vi "System Monitor.Async.vi"(10 "Parameters":variant, 11 "Process":refnum<class "Process.lvclass">) -> ()   [LabVIEW 2027, in "System Monitor Engine.lvlib"]
uses:
  System Monitor Engine.lvlib
  <vilib>/NI/NIVS Inline Async API/_VS Inline Async API/Process/Process.lvclass
  <vilib>/NI/NIVS Inline Async API/_VS Inline Async API/Process/Process.lvclass/Process.ctl
  Shared/Compiled.Settings.ctl
  Shared/System Monitor Settings.ctl
  <vilib>/Platform/TimedLoop/XDataNode/timing_clust.ctl
  <vilib>/Platform/TimedLoop/XDataNode/nitl_modes.ctl
  <vilib>/Platform/TimedLoop/XDataNode/wakeup.ctl
  <vilib>/NI/NIVS Inline Async API/_Data Access Engine/Access Type Classes/Write/Write.lvclass/Write.ctl
  <vilib>/NI/NIVS Inline Async API/_Data Access Engine/Data Access Engine/Methods/Write.Data.vi
  <vilib>/NI/NIVS Inline Async API/_VS Inline Async API/Error Handling Process/SubVIs/Error.ConvertArray.vi
  <vilib>/NI/NIVS Inline Async API/_Data Access Engine/Access Type Classes/Write/Write.ProcessData.vi
  <vilib>/NI/NIVS Inline Async API/_Data Access Engine/Access Type Classes/Write/Write.Buffer.vi
  <vilib>/NI/NIVS Inline Async API/_Data Access Engine/Access Type Classes/Write/Write.Commit.vi
  Shared/Constants.vi
  <vilib>/NI/NIVS Inline Async API/_Data Access Engine/Data Access Engine/Methods/Write.Lookup.vi
  <vilib>/NI/NIVS Inline Async API/_Data Access Engine/Data Access Engine/Data Access Engine.lvclass
  <vilib>/platform/TimedLoop/XDataNode/XDataNode.xnode
  Shared/System Monitor Shared.lvlib
  <vilib>/NI VeriStand/Custom Device Tools/Custom Device Utility Library/Custom Device Utility Library.lvlib
  <vilib>/Platform/TimedLoop/XDataNode/XDNodeRunTimeDep.lvlib
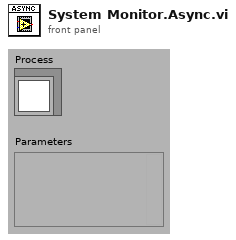
[diagram p1: front panel]
types:
  T1 = typedef "System Monitor Shared.lvlib/Compiled.Settings.ctl" = cluster{"Name":string, "System Monitor Settings":T2}
  T2 = typedef "System Monitor Shared.lvlib/System Monitor Settings.ctl" = cluster{"Number of CPU Cores":u64, "Update Rate (Hz)":dbl}
  T3 = typedef "Data Access Engine.lvlib/Data Access Engine.lvclass/Write.DVR.ctl" = refnum<data-value>
  T4 = typedef "XDNodeRunTimeDep.lvlib/timing_clust.ctl" = cluster{"Expected End [f-1]":u64, "Actual End [f-1]":u64, "Finished Late? [f-1]":bool, "Expected End [i-1]":u64, "Actual End [i-1]":u64, "Finished Late? [i-1]":bool, "Expected Start [i]":u64, "Actual Start [i]":u64, "Expected Start [f]":u64, "Actual Start [f]":u64, "Source Name":string, "Structure Name":string, "Period":i64, "Deadline":i64, "Offset":i64, "Start":i64, "Priority":i32, "Timeout":i32, "Mode":T5, "Wakeup Reason":T6, "Error":errorcluster, "Source Type":string, "Secondary Source Type":string, "Global End Time":u64, "Global Start Time":u64, "Frame Duration":u64, "Iteration Duration":u64, "Assigned CPU":i32, "I/O Scan Engine Mode":u32}
  T5 = typedef "XDNodeRunTimeDep.lvlib/nitl_modes.ctl" = enum32{"No Change", "Process missed periods, maintain original phase", "Discard missed periods, maintain original phase", "Process missed periods, ignore original phase", "Discard missed periods, ignore original phase"}
  T6 = typedef "XDNodeRunTimeDep.lvlib/wakeup.ctl" = enum32{"Normal", "Aborted", "Asynchronous wakeup", "Timing source error", "Timed loop error", "Timeout"}
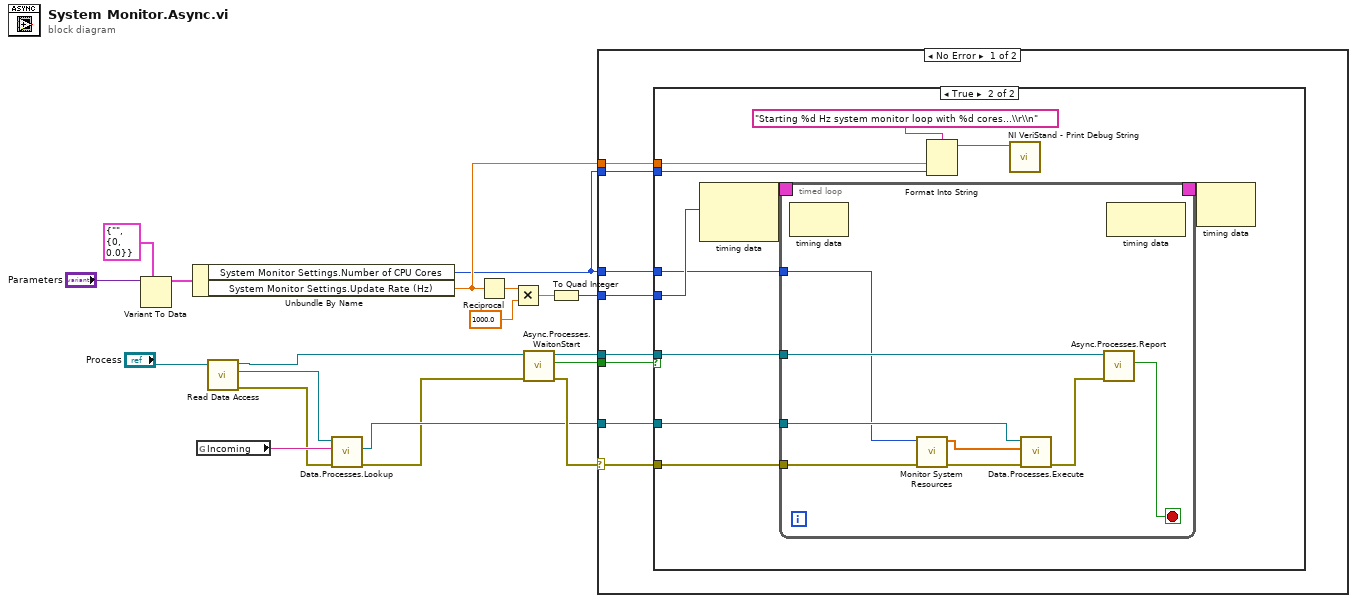
[diagram p0: block diagram]
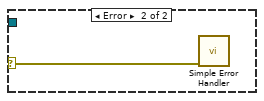
[diagram p3: hidden frame]
diagram:
  n1 = Variant To Data(type=T1 {"Name"="", "System Monitor Settings"={"Number of CPU Cores"=0, "Update Rate (Hz)"=0.0}} ("Compiled.Settings"), Variant="Parameters") -> (data=w13:T1)  [unwired: 1 in, 1 out]
  n2 = Unbundle By Name(w13) -> ("System Monitor Settings.Number of CPU Cores"=w6:u64, "System Monitor Settings.Update Rate (Hz)"=w7:dbl)
  n3 = global read "Constants.vi" "Incoming"() -> (w5:string)
  n4 = call <vilib>:"Read Data Access.vi"("Process in"="Process") -> ("error out"=w2:errorcluster, "Data Access"=w1:refnum<class "Data Access Engine.lvclass">, "Process out"=w3:refnum<class "Process.lvclass">)  [unwired: 8 in]
  n5 = call-poly <vilib>:"Data.Processes.Lookup.vi"("error in (no error)"=w2, "Name"=w5, "Data Access API in"=w1) -> ("error out"=w8:errorcluster, "Ref"=w16:T3)  [unwired: 5 in, 2 out]
  n6 = Reciprocal(x=w7) -> (1/x=w11:dbl)
  n7 = Multiply(x=w11, y=1000.0) -> (x*y=w10:dbl)
  n8 = call <vilib>:"Async.Processes.WaitonStart.vi"("error in (no error)"=w8, "Process"=w3) -> ("error out"=w17:errorcluster, "Execute"=w19:bool, "Process out"=w18:refnum<class "Process.lvclass">)  [unwired: 7 in]
  n9 = To Quad Integer(1:w10) -> (0:w9:i64)
  n10 = case shown="No Error" w17 {
    selector: w17 -> [w24 w53]
    tunnel: w19 -> [w27 _]
    tunnel: w18 -> [w26 _]
    tunnel: w16 -> [w25 _]
    tunnel: w9 -> [w23 _]
    tunnel: w6 -> [w22 _]
    tunnel: w7 -> [w21 _]
    tunnel: w6 -> [w20 _]
    frame No Error {
      n11 = case shown="True" w27 {
        tunnel: w24 -> [_ w36]
        tunnel: w26 -> [_ w37]
        tunnel: w25 -> [_ w38]
        tunnel: w23 -> [_ w31]
        tunnel: w22 -> [_ w30]
        tunnel: w21 -> [_ w29]
        tunnel: w20 -> [_ w28]
        frame False {
        }
        frame True {
          n12 = node-c288(w31) -> (w35:T4)  [unwired: 1 in]
          n13 = timed-loop {
            tunnel: w36 -> [w41]
            tunnel: w37 -> [w46]
            tunnel: w38 -> [w44]
            timing: w35 -> [_]
            timing-out: [_] -> w34
            tunnel: w30 -> [w42]
            stop <- w45 stop-if-true
            n14 = node-c288() -> ()  [unwired: 1 in, 1 out]
            n15 = call "Monitor System Resources.vi"("error in (no error)"=w41, "Number of CPU Cores"=w42) -> ("error out"=w40:errorcluster, "System Resources"=w39:dbl[])  [unwired: 8 in]
            n16 = call-poly <vilib>:"Data.Processes.Execute.vi"("error in (no error)"=w40, "Values"=w39, "Ref"=w44) -> ("error out"=w43:errorcluster)  [unwired: 8 in]
            n17 = call <vilib>:"Async.Processes.Report.vi"("Error"=w43, "Process in"=w46) -> ("Stop"=w45:bool)  [unwired: 8 in, 1 out]
            n18 = node-c288() -> ()  [unwired: 1 in, 1 out]
          }
          n19 = Format Into String(format string="Starting %d Hz system monitor loop with %d cores...\\r\\n", w29, w28) -> (resulting string=w33:string)  [unwired: 2 in, 1 out]
          n20 = call <vilib>:"NI VeriStand - Print Debug String.vi"("Message"=w33) -> ()  [unwired: 10 in, 1 out]
          n21 = node-c288(w34) -> ()  [unwired: 1 out]
        }
      }
    }
    frame Error {
      n22 = call <vilib>:"Simple Error Handler.vi"("error in (no error)"=w53) -> ()  [unwired: 4 in, 5 out]
    }
  }
